vi "Read Position Vector.vi"(8 "error in (no error)":errorcluster, 11 "Thruster in":refnum<class "Thruster.lvclass">) -> (0 "error out":errorcluster, 2 "Position Vector":dbl[](array[numeric]), 3 "Thruster out":refnum<class "Thruster.lvclass">)   [LabVIEW 2014, in "Thruster.lvclass"]
uses:
  Thruster.lvclass
  Thruster.lvclass/Thruster.ctl
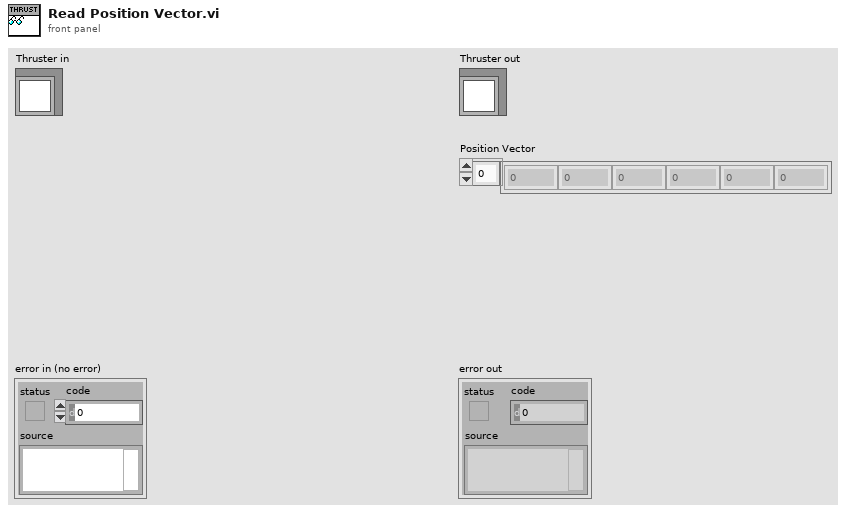
[diagram p1: front panel]
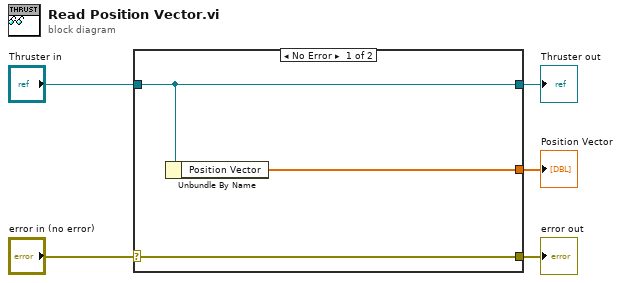
[diagram p0: block diagram]
diagram:
  n1 = case shown="No Error" "error in (no error)" {
    selector: "error in (no error)" -> [w8 w9]
    tunnel: [w8 w9] -> w4
    tunnel: [w7 w10] -> w2
    tunnel: "Thruster in" -> [w7 w10]
    tunnel: [w6 _] -> w1
    frame No Error {
      n2 = Unbundle By Name(w7) -> ("Position Vector"=w6:dbl[])
    }
    frame Error {
    }
  }
  "error out" <- w4
  "Thruster out" <- w2
  "Position Vector" <- w1
